vi "handleTermination.vi"(6 "timeout[ms]":i32, 8 "error in (no error)":errorcluster, 11 "TaskController in":refnum<class "TaskController.lvclass">) -> (0 "error out":errorcluster, 2 "terminated?":bool, 3 "TaskController out":refnum<class "TaskController.lvclass">)   [LabVIEW 2023, in "TLC_Daemon.lvlib" / "TaskController.lvclass"]
doc: "Waits for the task to terminate and executes all related cleanup and finalization operations."
uses:
  TaskController.lvclass
  TaskController.lvclass/TaskController.ctl
  ITask/ITask.lvclass
  ITaskChannel/ITaskChannel.lvclass
  status.ctl
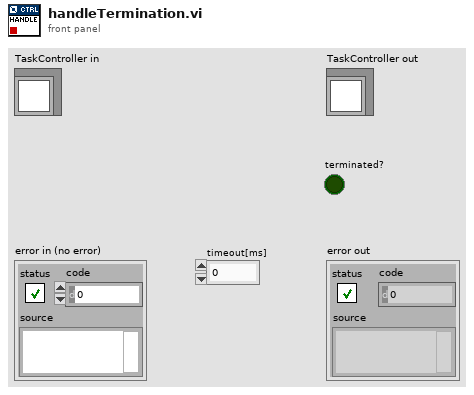
[diagram p1: front panel]
types:
  T1 = typedef "TLC_Daemon.lvlib/TaskController.lvclass/status.ctl" = enum16{"NotReady", "Ready", "Running", "Stopped", "Unknown"}
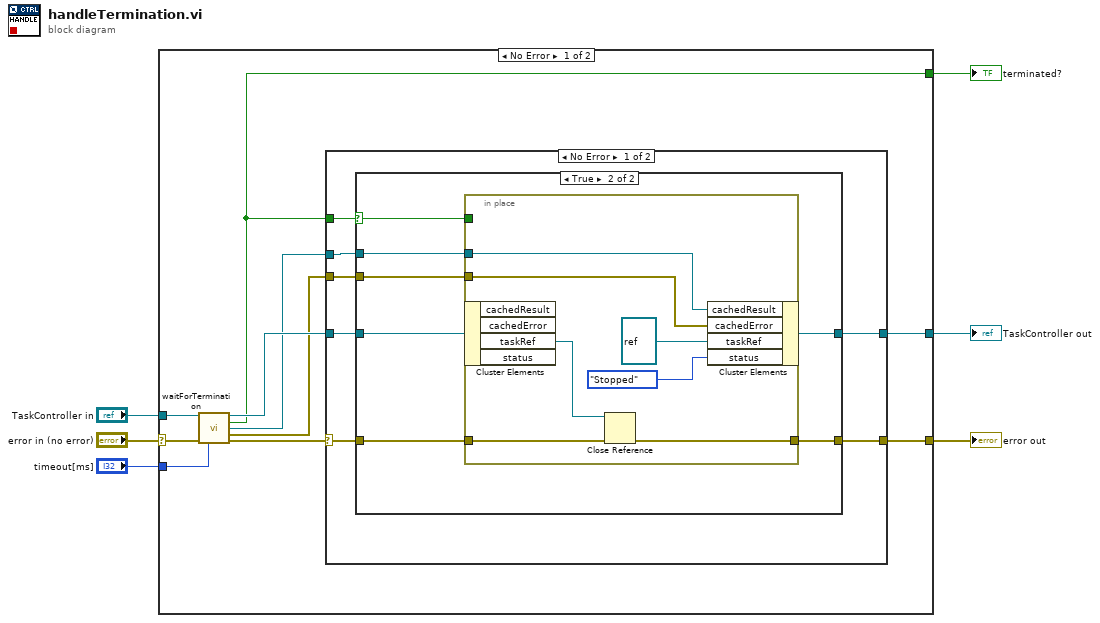
[diagram p0: block diagram]
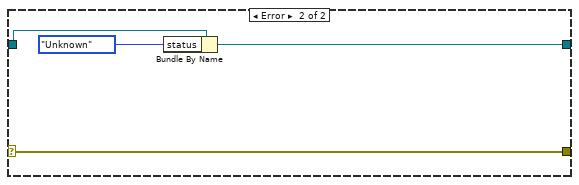
[diagram p3: hidden frame]
diagram:
  n1 = case shown="No Error" "error in (no error)" {
    selector: "error in (no error)" -> [w16 w45]
    tunnel: [w10 w45] -> w5
    tunnel: [w11 w44] -> w3
    tunnel: "TaskController in" -> [w13 w44]
    tunnel: "timeout[ms]" -> [w15 _]
    tunnel: [w7 _] -> w1
    frame No Error {
      n2 = call "waitForTermination.vi"("TaskController in"=w13, "error in (no error)"=w16, "timeout[ms]"=w15) -> ("TaskController out"=w12:refnum<class "TaskController.lvclass">, "terminated?"=w7:bool, "taskOut"=w9:refnum<class "ITask.lvclass">, "taskError"=w8:errorcluster, "error out"=w14:errorcluster)  [unwired: 8 in]
      n3 = case shown="No Error" w14 {
        selector: w14 -> [w18 w43]
        tunnel: w7 -> [w22 _]
        tunnel: w12 -> [w23 w42]
        tunnel: [w21 w41] -> w11
        tunnel: [w17 w43] -> w10
        tunnel: w9 -> [w20 _]
        tunnel: w8 -> [w19 _]
        frame No Error {
          n4 = case shown="True" w22 {
            selector: w22 -> [_ w30]
            tunnel: w23 -> [w25 w29]
            tunnel: [w25 w28] -> w21
            tunnel: w20 -> [_ w32]
            tunnel: w19 -> [_ w31]
            tunnel: w18 -> [w24 w27]
            tunnel: [w24 w26] -> w17
            frame False {
            }
            frame True {
              n5 = in-place {
                in-place-border: w32 -> [w39]
                in-place-border: w31 -> [w38]
                in-place-border: w30 -> [_]
                in-place-border: w27 -> [w35]
                in-place-border: [w34] -> w26
                n6 = in-place-cluster #1(w29) -> ("taskRef"=w36:refnum<vi>)  [unwired: 3 out]
                n7 = Close Reference(reference=w36, error in (no error)=w35) -> (error out=w34:errorcluster)
                n8 = in-place-cluster #1("cachedResult"=w39, "cachedError"=w38, "taskRef"=refnum<vi> refnum, "status"=status."Stopped") -> (w28:refnum<class "TaskController.lvclass">)
              }
            }
          }
        }
        frame Error {
          n9 = Bundle By Name(cluster=w42, "status"=status."Unknown") -> (w41:refnum<class "TaskController.lvclass">)
        }
      }
    }
    frame Error {
    }
  }
  "error out" <- w5
  "TaskController out" <- w3
  "terminated?" <- w1
